vi "Coordinate2Address.vi"(1 "Column":i32, 2 "Row":i32) -> (0 "Address":string)   [LabVIEW 2013, in "XCel Report Engine.lvlib"]
doc: "Converts zero-based row and column coordinates to an Excel A1 cell address.\n\nCoordinate (0, 0) returns A1. For example, row 12 and column 14 return O13.\n\nAn error is returned if either coordinate is negative or exceeds the Excel worksheet limits.\n\nThis conversion does not require an open report session."
uses:
  XCel Report Engine.lvlib
  C:/Users/m.santucci/Documents/ChatGPT/LV_REPORT_ENGINE/LV/DotNet/XCelReportEngine.dll
  LV/DotNet/XCelReportEngine.dll
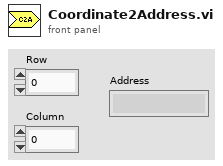
[diagram p1: front panel]
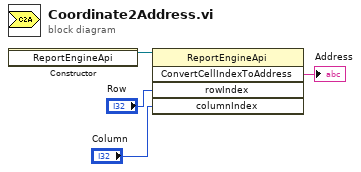
[diagram p0: block diagram]
diagram:
  n1 = constructor class="ReportEngineApi"() -> (reference out=w4:refnum<k24>)  [unwired: 3 in, 2 out]
  n2 = invoke class="ReportEngineApi" method="ConvertCellIndexToAddress"(reference=w4, "rowIndex"="Row", "columnIndex"="Column") -> ("ConvertCellIndexToAddress"=→"Address":string)  [unwired: 2 in, 4 out]
